vi "tagDB_Free.vi"(8 "error in (no error)":errorcluster, 11 "DB Ref":T1) -> (0 "error out":errorcluster)   [LabVIEW 2014, in "TagDB(dev).lvlib"]
doc: "[Covers: REQ_API_Free]"
uses:
  TagDB(dev).lvlib
  tagDB_Def.ctl
  _Support/Private/_DEF-DBOper.ctl
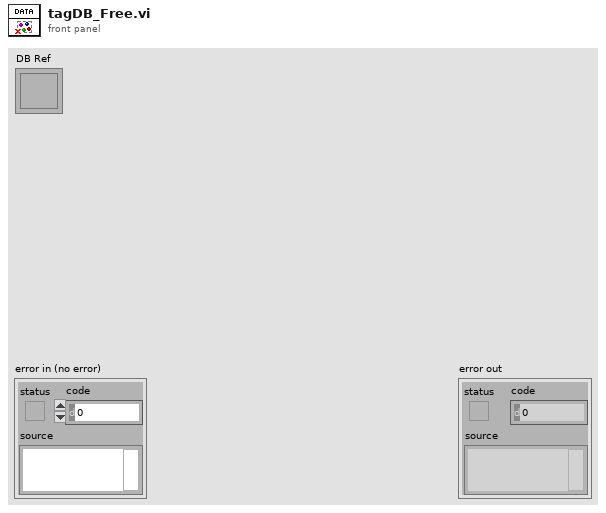
[diagram p1: front panel]
types:
  T1 = typedef "TagDB(dev).lvlib/tagDB_Def.ctl" = refnum<k1>
  T2 = typedef "TagDB(dev).lvlib/_DEF-DBOper.ctl" = enum16{"create", "destroy", "cleanUp", "list", "get info"}
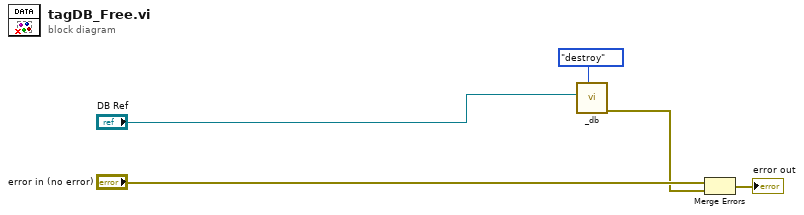
[diagram p0: block diagram]
diagram:
  n1 = call "_db.vi"("command"=_DEF-DBOper."destroy", "db in"="DB Ref") -> ("error out"=w2:errorcluster)  [unwired: 5 in, 4 out]
  n2 = Merge Errors("error in (no error)", w2) -> (→"error out":errorcluster)
